vi "Apply Velocity to Motors.vi"   [LabVIEW 2017, in "NI_Robotics_Steering Frame.lvclass"]
doc: "Calculates the velocity and angle of each motor necessary to satisfy the <B>steering frame velocity</B> or <B>arc velocity</B> at the center of a steering frame. You must manually select the polymorphic instance to use."
uses:
  <vilib>/robotics/Steering/Steering Frame/NI_Robotics_Steering Frame.lvclass
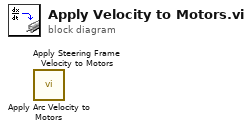
[diagram p0: block diagram]
diagram:
  n1 = call <vilib>:"Apply Arc Velocity to Motors.vi"() -> ()  [unwired: 7 in, 5 out]
  n2 = call <vilib>:"Apply Steering Frame Velocity to Motors.vi"() -> ()  [unwired: 7 in, 5 out]
